vi "response_stdfields.vi"(11 "HTTP Request":T1) -> (3 "HTTP Request out":T1)   [LabVIEW 2011]
uses:
  http_request_response.ctl
  http_request.ctl
  http_field.ctl
  http_response.ctl
  template_field.ctl
  template_field_type.ctl
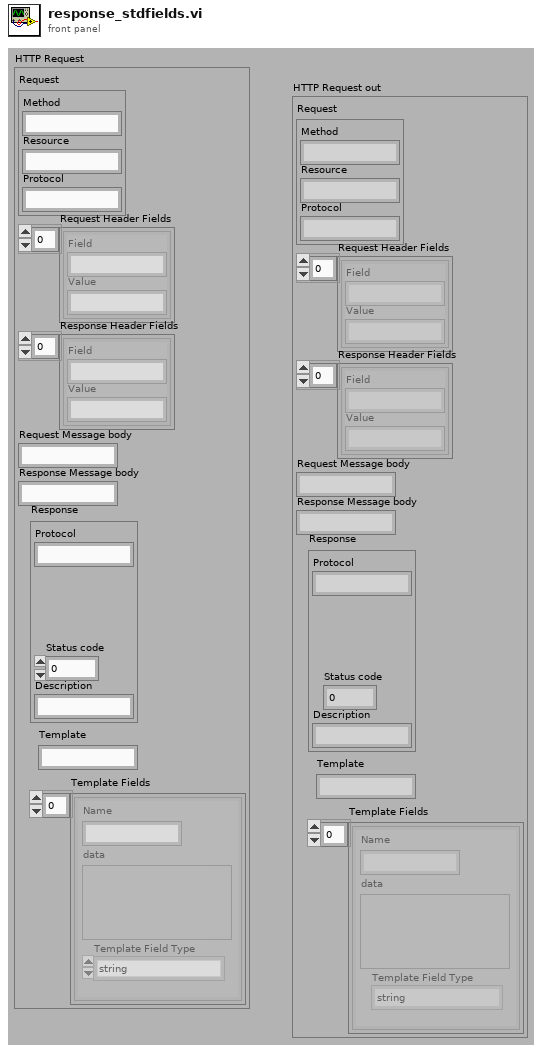
[diagram p1: front panel]
types:
  T1 = typedef "http_request_response.ctl" = cluster{"Request":T2, "Request Header Fields":T3[], "Response Header Fields":T3[], "Request Message body":string, "Response Message body":string, "Response":T4, "Template":string, "Template Fields":T5[]}
  T2 = typedef "http_request.ctl" = cluster{"Method":string, "Resource":string, "Protocol":string}
  T3 = typedef "http_field.ctl" = cluster{"Field":string, "Value":string}
  T4 = typedef "http_response.ctl" = cluster{"Protocol":string, "Status code":dbl, "Description":string}
  T5 = typedef "template_field.ctl" = cluster{"Name":string, "Template Field Type":T6, "data":variant}
  T6 = typedef "template_field_type.ctl" = enum16{"string", "string array", "number", "number array", "cluster", "cluster array"}
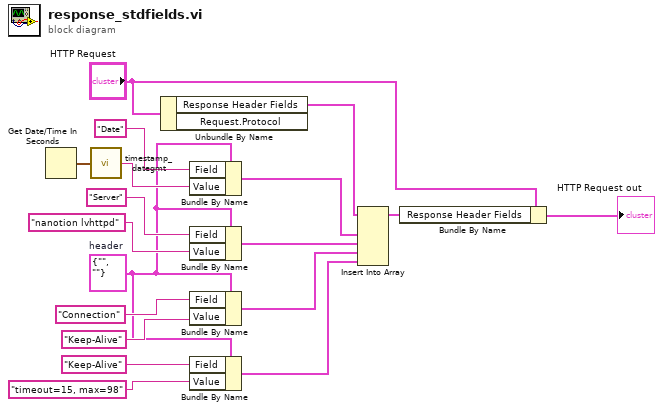
[diagram p0: block diagram]
diagram:
  w8 = T3 {"Field"="", "Value"=""}  # header
  n1 = Get Date/Time In Seconds() -> (seconds since 1Jan1904=w3:timestamp)
  n2 = call "timestamp_dategmt.vi"("time stamp"=w3) -> ("String"=w14:string)
  n3 = Unbundle By Name("HTTP Request") -> ("Response Header Fields"=w16:T3[])  [unwired: 1 out]
  n4 = Bundle By Name(cluster=w8, "Field"="Date", "Value"=w14) -> (w17:T3)
  n5 = Bundle By Name(cluster=w8, "Field"="Server", "Value"="nanotion lvhttpd") -> (w13:T3)
  n6 = Bundle By Name(cluster=w8, "Field"="Connection", "Value"="Keep-Alive") -> (w7:T3)
  n7 = Bundle By Name(cluster=w8, "Field"="Keep-Alive", "Value"="timeout=15, max=98") -> (w6:T3)
  n8 = Insert Into Array(array=w16, new element #1=w17, new element #2=w13, new element #3=w7, new element #4=w6) -> (w15:T3[])  [unwired: 1 in]
  n9 = Bundle By Name(cluster="HTTP Request", "Response Header Fields"=w15) -> (→"HTTP Request out":T1)
